vi "Timer with repeat.vi"() -> ()   [LabVIEW 2018]
panel:
  in  "stop":bool
  out "Remaining":u32
  in  "Number of Repeats":u32=3
  in  "Target Time (ms)":u32=3000
  out "Elapsed Time (ms)":u32
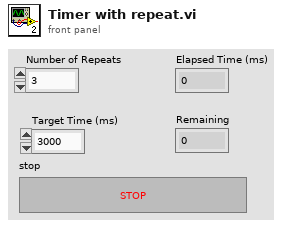
[diagram p1: front panel]
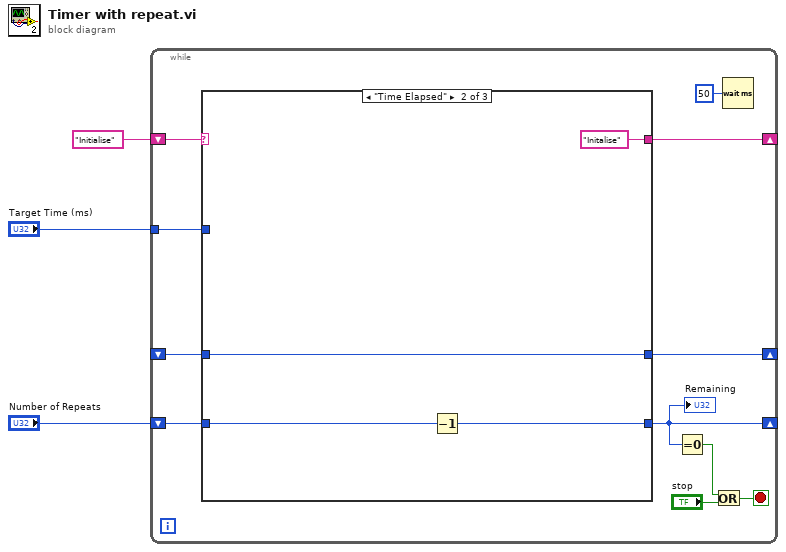
[diagram p0: block diagram]
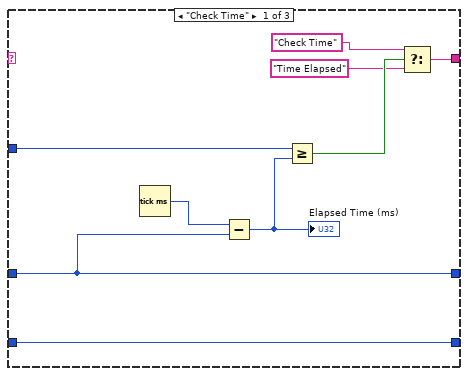
[diagram p2: hidden frame]
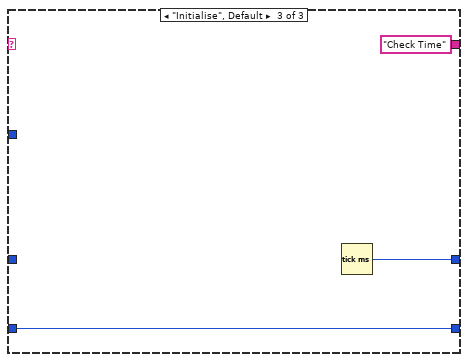
[diagram p3: hidden frame]
diagram:
  n1 = while {
    shift-right: [w13] -> _
    shift-left: _ -> [w11]
    shift-right: [w12] -> _
    shift-left: "Initialise" -> [w14]
    tunnel: "Target Time (ms)" -> [w10]
    shift-right: [w8] -> _
    shift-left: "Number of Repeats" -> [w9]
    stop <- w6 stop-if-true
    n2 = case shown="\"Time Elapsed\"" w14 {
      tunnel: [w22 w24 w30] -> w13
      tunnel: [w18 "Initalise" ("f") "Check Time"] -> w12
      tunnel: w11 -> [w22 w24 _]
      tunnel: w10 -> [w21 _ _]
      tunnel: w9 -> [w17 w27 w28]
      tunnel: [w17 w26 w28] -> w8
      frame "Check Time" {
        n3 = Tick Count (ms)() -> (millisecond timer value=w23:u32)
        n4 = Subtract(x=w23, y=w22) -> (x-y=w20:u32)
        "Elapsed Time (ms)" <- w20
        n5 = Greater Or Equal?(x=w21, y=w20) -> (x >= y?=w19:bool)
        n6 = Select(t="Check Time" ("f"), s=w19, f="Time Elapsed") -> (s? t:f=w18:string)
      }
      frame "Time Elapsed" {
        n7 = Decrement(x=w27) -> (x-1=w26:u32)
      }
      frame "Initialise", Default {
        n8 = Tick Count (ms)() -> (millisecond timer value=w30:u32)
      }
    }
    "Remaining" <- w8
    n9 = Equal To 0?(x=w8) -> (x = 0?=w7:bool)
    n10 = Or(x=w7, y="stop") -> (x .or. y?=w6:bool)
    n11 = Wait (ms)(milliseconds to wait=u32 50) -> ()  [unwired: 1 out]
  }
